vi "AddVirtualFolders.vi"(8 "error in (no error)":errorcluster) -> (0 "error out":errorcluster)   [LabVIEW 2013, in "ProjectHandler.lvlib"]
uses:
  ProjectHandler.lvlib
  RefNums.vi
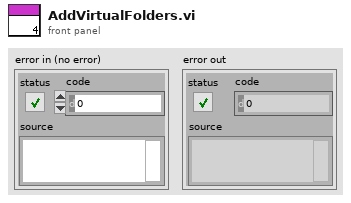
[diagram p1: front panel]
types:
  T1 = cluster{"App":refnum<vi>, "Project":refnum<vi>, "My Computer":refnum<vi>}
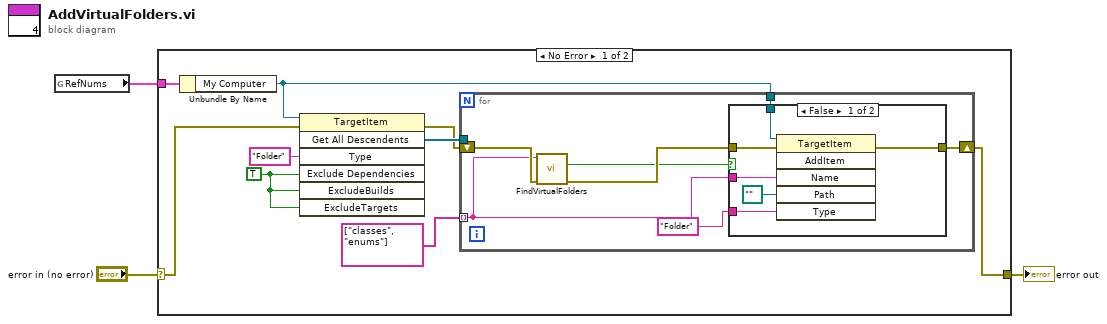
[diagram p0: block diagram]
diagram:
  n1 = global read "RefNums.vi" "RefNums"() -> (w1:T1)
  n2 = case shown="No Error" "error in (no error)" {
    selector: "error in (no error)" -> [w5 w27]
    tunnel: [w6 w27] -> w2
    tunnel: w1 -> [w12 _]
    frame No Error {
      w10 = TRUE ("ExcludeDependencies")
      n3 = Unbundle By Name(w12) -> ("My Computer"=w4:refnum<vi>)
      n4 = invoke class="TargetItem" method="Get All Descendents"(reference=w4, error in=w5, "Type"="Folder", "Exclude Dependencies"=w10, "ExcludeBuilds"=w10, "ExcludeTargets"=w10) -> (error out=w7:errorcluster, "All Descendents"=w8:refnum<vi>[])  [unwired: 1 in, 5 out]
      n5 = for {
        tunnel: string[] ["classes", "enums"] -> [w13] mode=indexing
        tunnel: w8 -> [_]
        shift-right: [w19] -> w6
        shift-left: w7 -> [w16]
        tunnel: w4 -> [w17]
        n6 = call "FindVirtualFolders.vi"("error in (no error)"=w16, "Name"=w13) -> ("error out"=w15:errorcluster, "Found"=w14:bool)  [unwired: 7 in, 1 out]
        n7 = case shown="False" w14 {
          tunnel: w15 -> [w25 w26]
          tunnel: [w24 w26] -> w19
          tunnel: w13 -> [w23 _]
          tunnel: "Folder" ("Type") -> [w21 _]
          tunnel: w17 -> [w20 _]
          frame False {
            n8 = invoke class="TargetItem" method="AddItem"(reference=w20, error in=w25, "Name"=w23, "Path"=path "", "Type"=w21) -> (error out=w24:errorcluster)  [unwired: 1 in, 5 out]
          }
          frame True {
          }
        }
      }
    }
    frame Error {
    }
  }
  "error out" <- w2
